vi "Empty and Restart FIFOs.vi"(8 "error in":errorcluster, 11 "FPGA VI Reference In":T1) -> (0 "error out":errorcluster, 3 "FPGA VI Reference Out":T1)   [LabVIEW 2017]
doc: "Author: Scott Hannahs <sth@magnet.fsu.edu>\nCopyright 2018 Florida State University, All rights reserved."
uses:
  RT Controls/FPGA SCH Digitizer Ref.ctl
  <vilib>/rvi/interface/nirviMethod/nirviMethod.xnode
  <vilib>/FPGAPlugInAG/Dynamic/niLvFpga_ReadFifo_Dynamic.vi
  <vilib>/rvi/errors/niLvFpgaMergeErrorWithErrorCode.vi
  <vilib>/FPGAPlugInAG/Dynamic/niLvFpga_StartFifo_Dynamic.vi
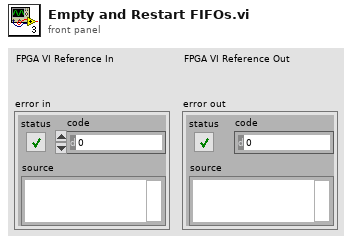
[diagram p1: front panel]
types:
  T1 = typedef "FPGA SCH Digitizer Ref.ctl" = refnum<k20>
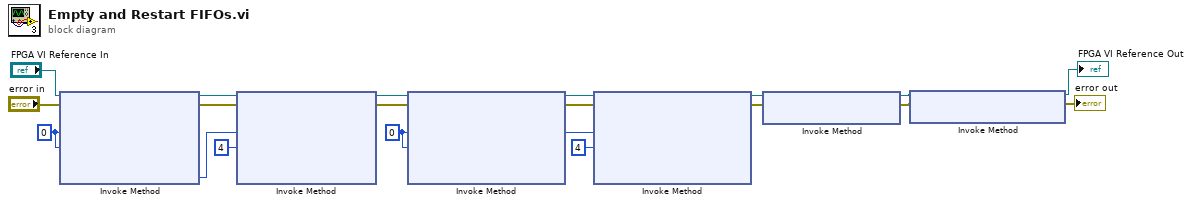
[diagram p0: block diagram]
diagram:
  w12 = u32 0 ("Number of Elements")
  w11 = u32 0 ("Number of Elements")
  n1 = xnode "Invoke Method"("FPGA VI Reference In"="FPGA VI Reference In", "error in"="error in", "Number of Elements"=w11, "Timeout (ms)"=w11) -> ("FPGA VI Reference Out"=w7:T1, "error out"=w14:errorcluster, "Elements Remaining"=w6:u32)  [unwired: 1 out]
  n2 = xnode "Invoke Method"("FPGA VI Reference In"=w7, "error in"=w14, "Number of Elements"=w6, "Timeout (ms)"=4) -> ("FPGA VI Reference Out"=w13:T1, "error out"=w15:errorcluster)  [unwired: 2 out]
  n3 = xnode "Invoke Method"("FPGA VI Reference In"=w13, "error in"=w15, "Number of Elements"=w12, "Timeout (ms)"=w12) -> ("FPGA VI Reference Out"=w8:T1, "error out"=w16:errorcluster, "Elements Remaining"=w9:u32)  [unwired: 1 out]
  n4 = xnode "Invoke Method"("FPGA VI Reference In"=w8, "error in"=w16, "Number of Elements"=w9, "Timeout (ms)"=4) -> ("FPGA VI Reference Out"=w19:T1, "error out"=w20:errorcluster)  [unwired: 2 out]
  n5 = xnode "Invoke Method"("FPGA VI Reference In"=w19, "error in"=w20) -> ("FPGA VI Reference Out"=w18:T1, "error out"=w17:errorcluster)
  n6 = xnode "Invoke Method"("FPGA VI Reference In"=w18, "error in"=w17) -> ("FPGA VI Reference Out"=→"FPGA VI Reference Out":T1, "error out"=→"error out":errorcluster)
